vi "人脸识别程序_2调用DB匹配.vi"(0 "分割后人脸图像":T1) -> (1 "识别结果":string, 2 "匹配图像":T1(plugin-control))   [LabVIEW 2017]
uses:
  <vilib>/vision/Image Controls.llb/IMAQ Image.ctl
  <vilib>/vision/NI_Vision_Development_Module.lvlib
panel:
  out "匹配图像路径":path
  out "Score":sgl
  out "识别成功":bool
  out "添加的路径":path
  out "Number of Matches":i32
  out "Matches (pixel)":T2(array[cluster]) {"Bounding Box"."y" format="%.2f"; "Bounding Box"."x" format="%.2f"; "Score" format="%.2f"; "Scale" format="%.2f"; "Angle" format="%.2f"; "Position"."y" format="%.2f"; "Position"."x" format="%.2f"}
  out "模板图像":T1(plugin-control)
  in  "人脸DB基路径":path=path "D:/机器视觉_短学期/课程项目/人脸图像DB"
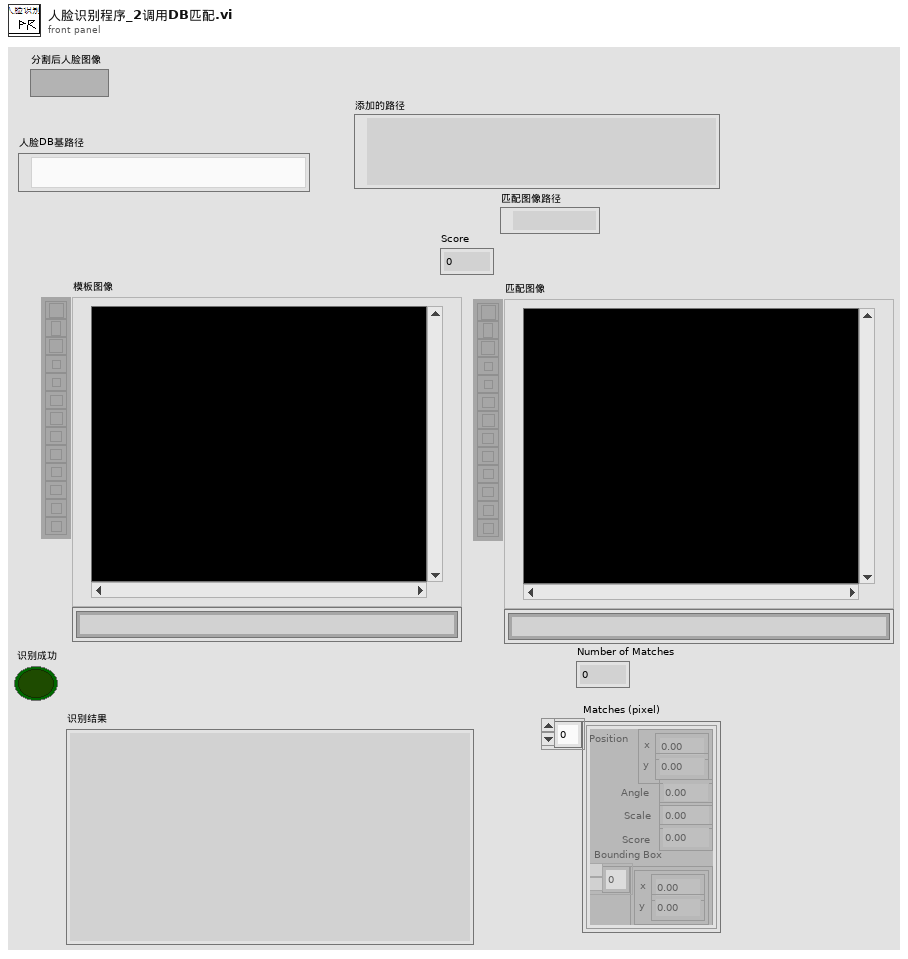
[diagram p1: front panel]
types:
  T1 = typedef "IMAQ Image.ctl" = refnum<image>
  T2 = cluster{"Position":cluster{"x":sgl, "y":sgl}, "Angle":sgl, "Scale":sgl, "Score":sgl, "Bounding Box":cluster{"x":sgl, "y":sgl}[]}[]
  T3 = typedef "Image Type" = u32
  T4 = cluster{"Position":cluster{"x":sgl, "y":sgl}, "Angle":sgl, "Scale":sgl, "Score":sgl, "Bounding Box":cluster{"x":sgl, "y":sgl}[]}
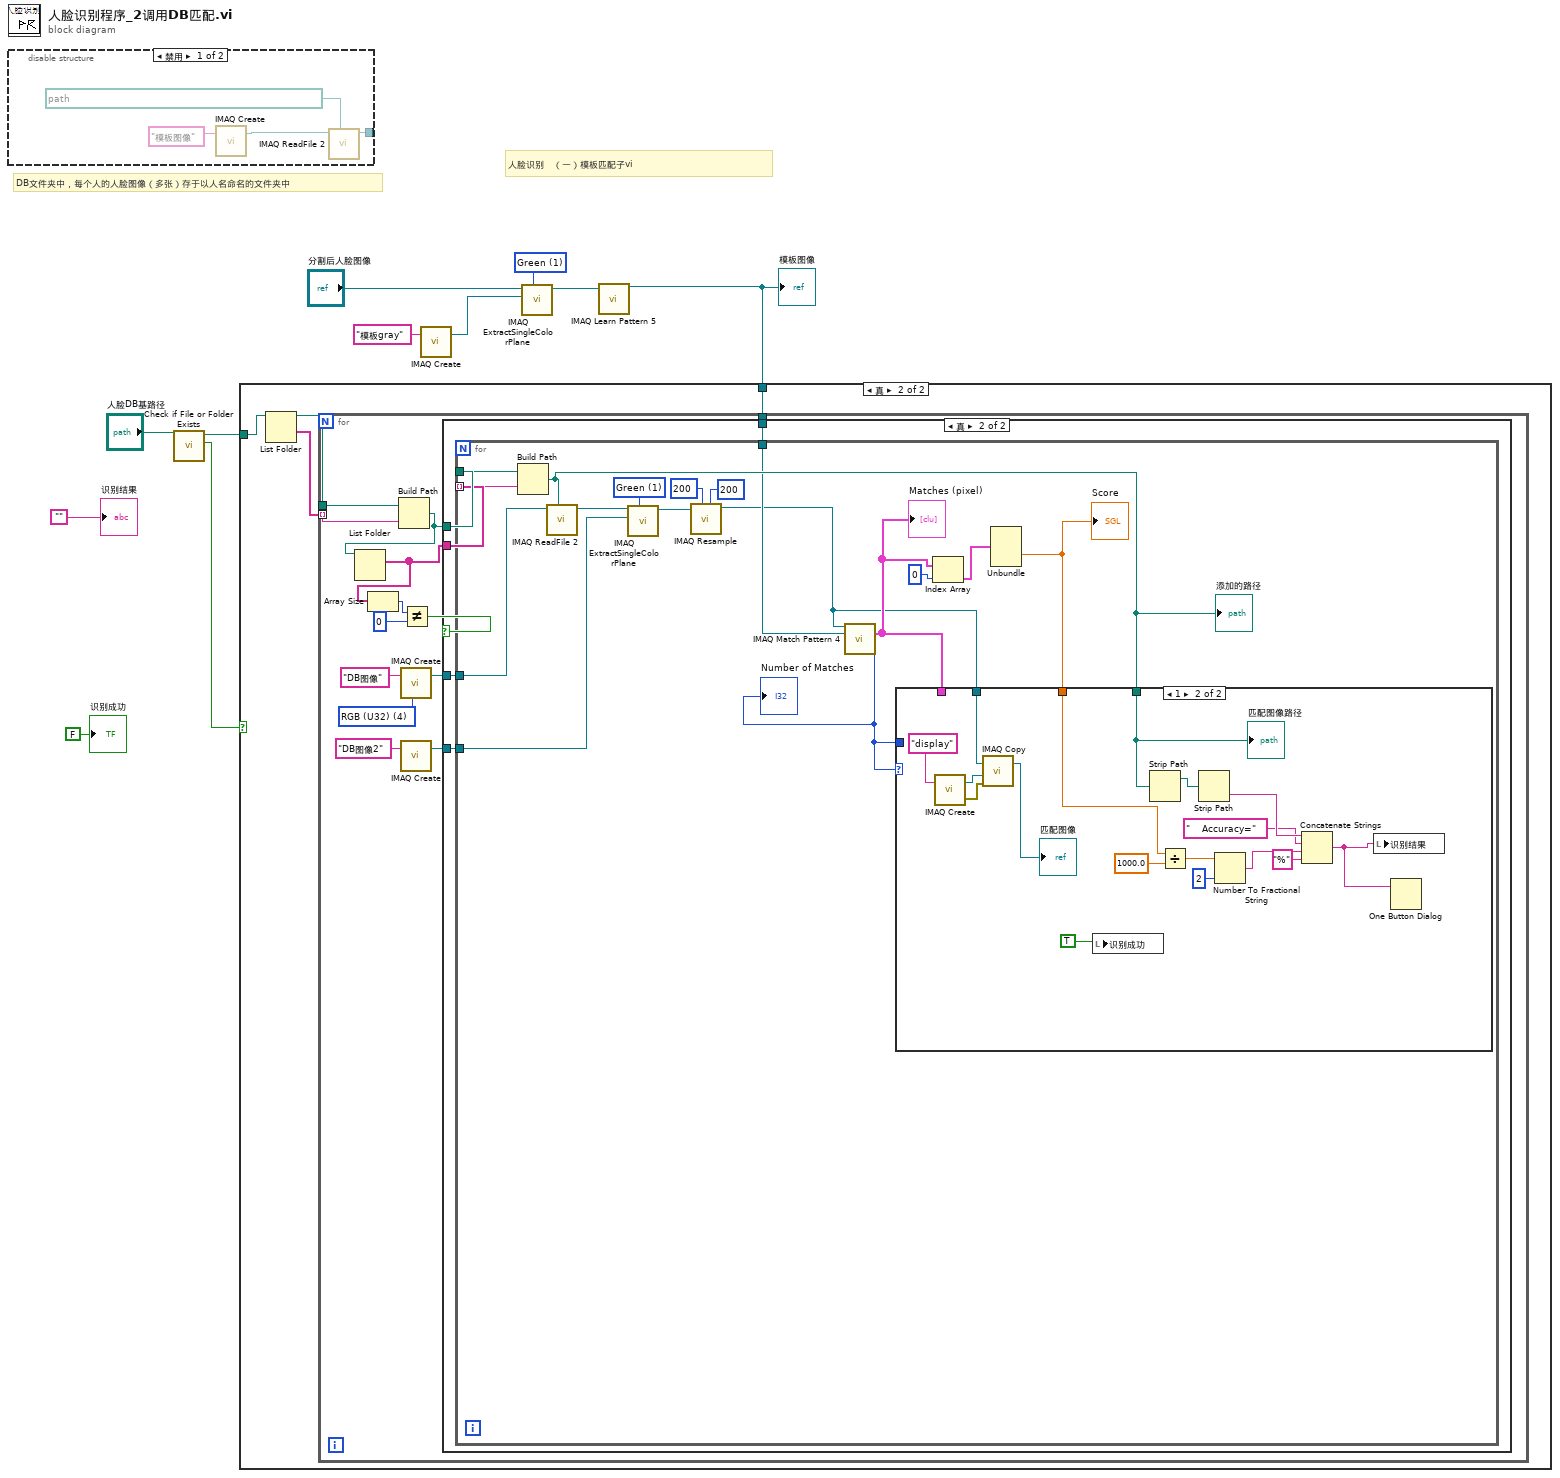
[diagram p0: block diagram]
diagram:
  w8 = 1 items=["Red", "Green", "Blue", "Hue", "Saturation", "Luminance", "Value", "Intensity"] ("Color Plane")
  # "人脸识别   （一）模板匹配子vi"
  # "DB文件夹中，每个人的人脸图像（多张）存于以人名命名的文件夹中"
  n1 = disable-structure shown="禁用" {
    disable-tunnel: [w12 _] -> _
    frame Disabled {
      n2 = call "IMAQ Create"("Image Name"="模板图像") -> ("New Image"=w13:T1)  [unwired: 4 in, 1 out]
      n3 = call "IMAQ ReadFile 2"("File Path"=path "D:/机器视觉_短学期/课程项目/人脸图像DB/5.jpg", "Image"=w13) -> ("Image Out"=w12:T1)  [unwired: 5 in, 4 out]
    }
    frame Enabled {
    }
  }
  n4 = call <vilib>:"Check if File or Folder Exists.vi"("path"="人脸DB基路径") -> ("file or folder exists?"=w10:bool, "dup path"=w9:path)  [unwired: 8 in, 1 out]
  n5 = call "IMAQ Create"("Image Name"="模板gray") -> ("New Image"=w2:T1)  [unwired: 4 in, 1 out]
  n6 = call "IMAQ ExtractSingleColorPlane"("Color Plane"=w8, "Image Dst"=w2, "Image Src"="分割后人脸图像") -> ("Image Dst Out"=w7:T1)  [unwired: 7 in, 1 out]
  n7 = call "IMAQ Learn Pattern 5"("Image"=w7) -> ("Template Image Out"=w6:T1)  [unwired: 12 in, 2 out]
  "模板图像" <- w6
  n8 = case shown="真" w10 {
    tunnel: w9 -> [_ w19]
    tunnel: w6 -> [_ w16]
    frame False {
    }
    frame True {
      n9 = List Folder(path=w19) -> (path out=w18:path, folder names=w17:string[])  [unwired: 3 in, 2 out]
      n10 = for {
        tunnel: w17 -> [w32] mode=indexing
        tunnel: w18 -> [w26]
        tunnel: w16 -> [w20]
        w24 = T3 4 items=["Grayscale (U8)", "Grayscale (I16)", "Grayscale (SGL)", "Complex (CSG)", "RGB (U32)", "HSL (U32)", "RGB (U64)", "Grayscale (U16)"] ("Image Type")
        n11 = Build Path(base path=w26, name or relative path=w32) -> (appended path=w28:path)
        n12 = List Folder(path=w28) -> (filenames=w27:string[])  [unwired: 3 in, 3 out]
        n13 = Array Size(array=w27) -> (size(s)=w31:i32)
        n14 = call "IMAQ Create"("Image Name"="DB图像", "Image Type"=w24) -> ("New Image"=w23:T1)  [unwired: 3 in, 1 out]
        n15 = call "IMAQ Create"("Image Name"="DB图像2") -> ("New Image"=w21:T1)  [unwired: 4 in, 1 out]
        n16 = Not Equal?(x=w31, y=0) -> (x != y?=w29:bool)
        n17 = case shown="真" w29 {
          tunnel: w28 -> [_ w37]
          tunnel: w27 -> [_ w36]
          tunnel: w23 -> [_ w35]
          tunnel: w21 -> [_ w34]
          tunnel: w20 -> [_ w33]
          frame False {
          }
          frame True {
            n18 = for {
              tunnel: w37 -> [w54]
              tunnel: w36 -> [w53] mode=indexing
              tunnel: w35 -> [w52]
              tunnel: w34 -> [w50]
              tunnel: w33 -> [w45]
              w49 = 1 items=["Red", "Green", "Blue", "Hue", "Saturation", "Luminance", "Value", "Intensity"] ("Color Plane")
              n19 = Build Path(base path=w54, name or relative path=w53) -> (appended path=w46:path)
              "添加的路径" <- w46
              n20 = call "IMAQ ReadFile 2"("File Path"=w46, "Image"=w52) -> ("Image Out"=w51:T1)  [unwired: 5 in, 4 out]
              n21 = call "IMAQ ExtractSingleColorPlane"("Color Plane"=w49, "Image Dst"=w50, "Image Src"=w51) -> ("Image Dst Out"=w39:T1)  [unwired: 7 in, 1 out]
              n22 = call "IMAQ Resample"("X Resolution"=200, "Y Resolution"=200, "Image Src"=w39) -> ("Image Dst Out"=w38:T1)  [unwired: 7 in, 1 out]
              n23 = call "IMAQ Match Pattern 4"("Image"=w38, "Template Image"=w45) -> ("Matches (pixel)"=w44:T2, "Number of Matches"=w43:i32)  [unwired: 9 in, 3 out]
              "Matches (pixel)" <- w44
              "Number of Matches" <- w43
              n24 = Index Array(array=w44, index=0 ("索引")) -> (element=w47:T4)
              n25 = Unbundle(w47) -> ("Score"=w42:sgl)  [unwired: 4 out]
              "Score" <- w42
              n26 = case shown="1" w43 {
                tunnel: w46 -> [_ w63]
                tunnel: w43 -> [_ _]
                tunnel: w44 -> [_ _]
                tunnel: w42 -> [_ w61]
                tunnel: w38 -> [_ w60]
                frame 0, Default {
                }
                frame 1 {
                  n27 = call "IMAQ Create"("Image Name"="display") -> ("New Image"=w59:T1, "error out"=w58:errorcluster)  [unwired: 4 in]
                  n28 = call "IMAQ Copy"("error in (no error)"=w58, "Image Dst"=w59, "Image Src"=w60) -> ("Image Dst Out"=→"匹配图像":T1)  [unwired: 3 in, 1 out]
                  n29 = local write "识别成功"(TRUE) -> ()
                  n30 = Strip Path(path=w63) -> (stripped path=w68:path)  [unwired: 1 out]
                  n31 = Divide(x=w61, y=sgl 1000.0) -> (x/y=w69:sgl)
                  n32 = Strip Path(path=w68) -> (name=w70:string)  [unwired: 1 out]
                  n33 = Number To Fractional String(number=w69, precision (6)=i16 2 ("精度(6)")) -> (F-format string=w71:string)  [unwired: 2 in]
                  n34 = Concatenate Strings(w70, "    Accuracy=" ("字符串"), w71, "%" ("字符串")) -> (w55:string)
                  n35 = local write "识别结果"(w55) -> ()
                  n36 = One Button Dialog(message=w55) -> ()  [unwired: 1 in, 1 out]
                  "匹配图像路径" <- w63
                }
              }
            }
          }
        }
      }
    }
  }
  "识别结果" <- ""
  "识别成功" <- FALSE ("识别成功")
